vi "SetFs.vi"(8 "error in (no error)":errorcluster, 9 "Fs":dbl format="%#_6pHz", 10 "Port":string(combo), 11 "reference in":refnum<class "sim_MmW.lvclass">) -> (0 "error out":errorcluster, 3 "reference out":refnum<class "sim_MmW.lvclass">)   [LabVIEW 2019, in "sim_MmW.lvclass"]
doc: "Set sampling frequency for port"
uses:
  sim_MmW.lvclass
  mmWave instrument_class/mmWave instrument.lvclass
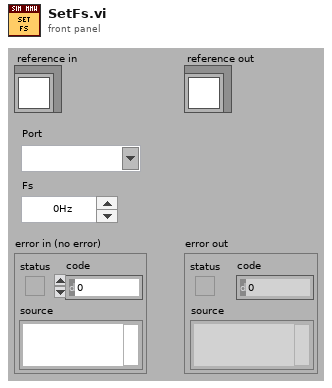
[diagram p1: front panel]
types:
  T1 = typedef "sim_MmW.lvclass/ObjectAttributesRef.ctl" = refnum<data-value>
  T2 = typedef "sim_MmW.lvclass/ObjectAttributes.ctl" = cluster{"RF config":T3, "RX samples":i32, "Downloaded Bursts":map{string, refnum<class "mmWave data.lvclass">}, "TX Fs":dbl, "RX Fs":dbl, "burst sequence":string[], "Burst mode":T4}
  T3 = typedef "mmWave HW Control.lvlib/HW TXRX RF config cluster.ctl" = cluster{"TX.Frequency":dbl, "TX.Gain":dbl, "TX.mmWave adapter":string, "RX.Frequency":dbl, "RX.Gain":dbl, "RX.mmWave adapter":string}
  T4 = typedef "mmWave instrument.lvclass/BurstMode.ctl" = enum16{"burst", "continuous"}
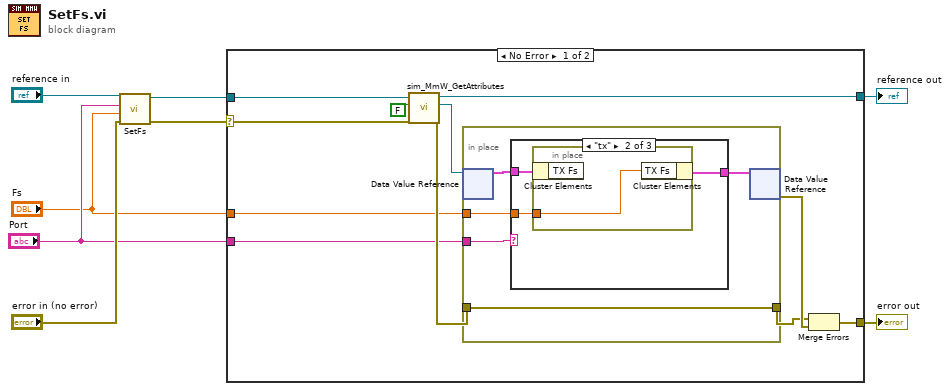
[diagram p0: block diagram]
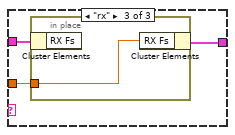
[diagram p3: hidden frame]
diagram:
  n1 = call-parent "SetFs.vi"("error in (no error)"="error in (no error)", "Fs"="Fs", "Port"="Port", "reference in"="reference in") -> ("error out"=w5:errorcluster, "reference out"=w4:refnum<class "sim_MmW.lvclass">)  [unwired: 6 in]
  n2 = case shown="No Error" w5 {
    selector: w5 -> [w12 w34]
    tunnel: [w19 w34] -> w8
    tunnel: [w14 w35] -> w6
    tunnel: w4 -> [w11 w35]
    tunnel: "Port" -> [w10 _]
    tunnel: "Fs" -> [w9 _]
    frame No Error {
      n3 = call "sim_MmW_GetAttributes.vi"("error in (no error)"=w12, "return data? (T)"=FALSE, "reference in"=w11) -> ("error out"=w15:errorcluster, "attributes ref"=w13:T1, "reference out"=w14:refnum<class "sim_MmW.lvclass">)  [unwired: 5 in, 1 out]
      n4 = in-place {
        in-place-border: w15 -> [w22]
        in-place-border: [w22] -> w17
        in-place-border: w10 -> [w21]
        in-place-border: w9 -> [w20]
        n5 = in-place-dvr #1(w13) -> (w23:T2)  [unwired: 1 out]
        n6 = case shown="\"tx\"" w21 {
          tunnel: [w25 w28 w32] -> w24
          tunnel: w23 -> [w25 w27 w31]
          tunnel: w20 -> [_ w26 w30]
          frame "False", Default {
          }
          frame "tx" {
            n7 = in-place {
              in-place-border: w26 -> [w29]
              n8 = in-place-cluster #2(w27) -> ()  [unwired: 1 out]
              n9 = in-place-cluster #2("TX Fs"=w29) -> (w28:T2)
            }
          }
          frame "rx" {
            n10 = in-place {
              in-place-border: w30 -> [w33]
              n11 = in-place-cluster #3(w31) -> ()  [unwired: 1 out]
              n12 = in-place-cluster #3("RX Fs"=w33) -> (w32:T2)
            }
          }
        }
        n13 = in-place-dvr #1(w24) -> (w18:errorcluster)  [unwired: 1 out]
      }
      n14 = Merge Errors(w17, w18) -> (w19:errorcluster)
    }
    frame Error {
    }
  }
  "error out" <- w8
  "reference out" <- w6
